vi "Make Request.vi"(8 "error in (no error)":errorcluster, 11 "Session in":refnum<class "Session.lvclass">) -> (0 "error out":errorcluster, 2 "Response":T1, 3 "Session out":refnum<class "Session.lvclass">)   [LabVIEW 2015, in "NI_Azure_Blob.lvlib"]
doc: "This core implementation of Azure HTTP requests may be used to implement special requests or API calls not present in this toolkit."
uses:
  NI_Azure_Blob.lvlib
  Core/Session/Session.lvclass
  Core/Response.ctl
  Core/Session/Session.lvclass/Session.ctl
  Core/Session/Write _ServiceName.vi
  Core/NI_Azure_Core.lvlib
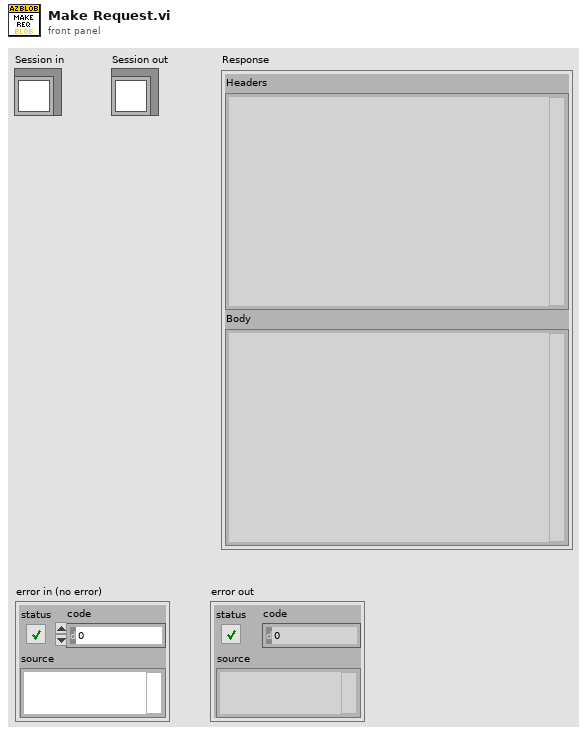
[diagram p1: front panel]
types:
  T1 = typedef "NI_Azure_Core.lvlib/Response.ctl" = cluster{"Headers":string, "Body":string}
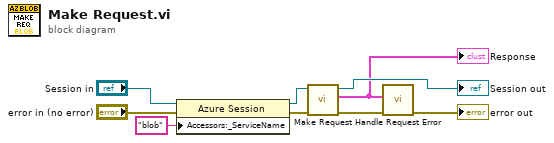
[diagram p0: block diagram]
diagram:
  n1 = property class="Azure Session"(reference="Session in", error in="error in (no error)", "Accessors:_ServiceName"="blob" ("_ServiceName")) -> (reference out=w2:refnum<class "Session.lvclass">, error out=w4:errorcluster)
  n2 = call "Make Request.vi"("error in (no error)"=w4, "Session in"=w2) -> ("error out"=w9:errorcluster, "Response"=w5:T1, "Session out"=→"Session out":refnum<class "Session.lvclass">)  [unwired: 7 in]
  "Response" <- w5
  n3 = call "Handle Request Error.vi"("error in (no error)"=w9, "Response"=w5) -> ("error out"=→"error out":errorcluster)  [unwired: 9 in]
